vi "UHR-Fleezers Control (host) - 10.8.vi"() -> ()   [LabVIEW 2014] (continued)
    n2212 = Cluster To Array(cluster=w3125) -> (array=w3122:string[])
    n2213 = Bundle("APD 1", "APD 2") -> (w3310:cluster{string, string})  [unwired: 1 out]
    n2214 = Select(t=-1.0, s="Negate Y Axis", f=1.0) -> (s? t:f=w3066:dbl)
    n2215 = for "Trap Position" {
      tunnel: w3131 -> [w3506] mode=indexing
      tunnel: "Trap Pos. Disp. Downsample" -> [w3505]
      tunnel: w3047 -> [w3503]
      tunnel: w3127 -> [w3502]
      tunnel: w3126 -> [w3500]
      tunnel: w3122 -> [w3499] mode=indexing
      tunnel: [w3498] -> w3036 mode=indexing
      tunnel: w3081 -> [w3496] mode=indexing
      tunnel: w3080 -> [w3494]
      tunnel: w3066 -> [w3493]
      n2216 = call "downsample 1D array - double.vi"("Ave N"=w3505, "Array In"=w3506) -> ("Array Out"=w3504:dbl[])  [unwired: 1 out]
      n2217 = Subtract(x=w3504, y=w3496) -> (x-y=w3497:dbl[])
      n2218 = Multiply(x=w3494, y=w3497) -> (x*y=w3495:dbl[])
      n2219 = Multiply(x=w3493, y=w3495) -> (x*y=w3492:dbl[])
      n2220 = Bundle By Name("Y"=w3492, "dt"=w3503, "t0"=w3502) -> (w3501:waveform(dbl))  [unwired: 1 out]
      n2221 = Set Waveform Attribute(5:w3499, 6:w3500, 7:w3501) -> (3:w3498:waveform(dbl))  [unwired: 1 in, 2 out]
    }
    n2222 = Cluster To Array(cluster=w3310) -> (array=w3307:string[])
    n2223 = for "APD" {
      tunnel: w3278 -> [w3846] mode=indexing
      tunnel: w3156 -> [w3854]
      tunnel: [w3850] -> w3163 mode=indexing
      tunnel: "APD Disp. Scale" -> [w3851]
      tunnel: w3126 -> [w3849]
      tunnel: w3307 -> [w3848] mode=indexing
      tunnel: "APD Disp. Downsample" -> [w3844]
      tunnel: [w3847] -> w3306
      workers-P: _ -> [_]
      tunnel: w3127 -> [w3843]
      n2224 = call "integrate 1D array interval - double.vi"("Ave N"=w3844, "Array In"=w3846) -> ("Array Out"=w3845:dbl[])  [unwired: 1 out]
      n2225 = Multiply(x=w3854, y=w3844) -> (x*y=w3847:dbl)
      n2226 = Divide(x=w3845, y=w3851) -> (x/y=w3852:dbl[])
      n2227 = Bundle By Name("t0"=w3843, "Y"=w3852, "dt"=w3847) -> (w3853:waveform(dbl))  [unwired: 1 out]
      n2228 = Set Waveform Attribute(5:w3848, 6:w3849, 7:w3853) -> (3:w3850:waveform(dbl))  [unwired: 1 in, 2 out]
    }
    "APD Display Period (s)" <- w3306
    n2229 = Reciprocal(x=w3306) -> (1/x=→"APD Display Freq. (Hz)":dbl)
    n2230 = local read "Display Period (s)"() -> (w3187:dbl)
    n2231 = Increment(x=w3289) -> (x+1=w3290:dbl)
    n2232 = To Double Precision Float(number=w3199) -> (double precision float=w3198:dbl[])
    n2233 = Index Array(array=w3036, index=0) -> (element=w3040:waveform(dbl))
    n2234 = Index Array(array=w3036, index=1) -> (element=w3035:waveform(dbl))
    n2235 = feedback #7(w3290) -> (w3293:dbl)
    n2236 = Select(t=0, s=w3280, f=w3293) -> (s? t:f=w3286:dbl)
    n2237 = Array Size(array=w3198) -> (size(s)=w3292:i32)
    n2238 = Add(x=w3292, y=w3286) -> (x+y=w3287:dbl)
    n2239 = Unbundle By Name(w3040) -> ("Y"=w3041:dbl[])
    n2240 = feedback #8(w3199) -> (w3276:void[])
    n2241 = Build Array (concatenate)(w3276, w3199) -> (w3273:void[])
    n2242 = feedback #9(w3143) -> (w3162:void[])
    n2243 = Divide(x="Bead Sep. Int. Time (s)", y=w3187) -> (x/y=w3076:dbl)
    n2244 = Build Array (concatenate)(w3162, w3143) -> (w3161:void[])
    n2245 = Add(x=w3041, y="FB Trap Pos Offset") -> (x+y=w3039:dbl[])
    "T1 x pos data" <- w3039
    n2246 = Greater?(x=w3287, y=w3289) -> (0:w3288:bool)
    n2247 = feedback #10(w3039) -> (w3078:dbl[])
    n2248 = Build Array (concatenate)(w3039, w3078) -> (w3077:dbl[])
    n2249 = Bundle By Name(cluster=w3040, "Y"=w3039) -> (w3038:waveform(dbl))
    n2250 = Select(t=w3286, s=w3288, f=w3287) -> (s? t:f=w3285:dbl)
    n2251 = feedback-in #7(w3285) -> ()
    n2252 = Array Size(array=w3273) -> (size(s)=w3270:i32)
    n2253 = Array Size(array=w3199) -> (size(s)=w3272:i32)
    n2254 = local read "MCL Scanning"() -> (w3283:bool)
    n2255 = local read "APD Integration Time (s)"() -> (w3170:dbl)
    n2256 = Bundle(w3038, w3035) -> (w3034:cluster{waveform(dbl), waveform(dbl)})  [unwired: 1 out]
    n2257 = Build Array (concatenate)(w3163, w3311) -> (w3165:waveform(dbl)[])
    "All Signals" <- w3165
    n2258 = Split 1D Array(array=w3077, index=w3076) -> (first subarray=w3070:dbl[])  [unwired: 1 out]
    n2259 = feedback-in #10(w3070) -> ()
    n2260 = Multiply(x=w3272, y="APD Ave N") -> (x*y=w3271:dbl)
    n2261 = Greater?(x=w3270, y=w3271) -> (0:w3274:bool)
    n2262 = Not(x=w3288) -> (.not. x?=w3282:bool)
    n2263 = Cluster To Array(cluster=w3034) -> (array=→"Trap Positions":waveform(dbl)[])
    n2264 = To Double Precision Float(number=w3143) -> (double precision float=w3142:dbl[])
    n2265 = call-poly <vilib>:"Mean.vi"("X"=w3070) -> ("mean"=w3069:dbl)  [unwired: 1 out]
    "Mean T1 Position (nm)" <- w3069
    n2266 = Subtract(x=w3070, y=w3069) -> (x-y=w3075:dbl[])
    n2267 = Square(x=w3075) -> (x^2=w3074:dbl[])
    n2268 = And(x=w3282, y=w3283) -> (x .and. y?=w3284:bool)
    n2269 = call-poly <vilib>:"Mean.vi"("X"=w3074) -> ("mean"=w3073:dbl)  [unwired: 1 out]
    n2270 = case shown="True" w3274 {
      tunnel: w3273 -> [w3626 w3633]
      tunnel: [w3626 w3631] -> w3216
      tunnel: w3271 -> [_ w3628]
      tunnel: w3270 -> [_ w3632]
      tunnel: w3161 -> [w3625 w3630]
      tunnel: [w3625 w3627] -> w3158
      frame False {
      }
      frame True {
        n2271 = Subtract(x=w3632, y=w3628) -> (x-y=w3629:dbl)
        n2272 = Array Subset(array=w3633, index=w3629, length=w3628) -> (w3631:void[])
        n2273 = Array Subset(array=w3630, index=w3629, length=w3628) -> (w3627:void[])
      }
    }
    n2274 = feedback-in #8(w3216) -> ()
    n2275 = feedback-in #9(w3158) -> ()
    n2276 = Square Root(x=w3073) -> (sqrt(x)=w3072:dbl)
    n2277 = Or(x=w3284, y=w3280) -> (x .or. y?=w3281:bool)
    n2278 = Equal?(x="Tab Control 6", y=T34."High Res Display") -> (x = y?=w3205:bool)
    n2279 = Multiply(x="APD Disp. Scale", y=w3163) -> (x*y=w3172:waveform(dbl)[])
    n2280 = Multiply(x=10.0, y=w3072) -> (x*y=→"Trap 1 Position RMS (A)":dbl)
    n2281 = Multiply(x="APD Disp. Downsample", y=w3170) -> (x*y=w3168:dbl)
    n2282 = Divide(x=w3172, y=w3168) -> (x/y=w3140:waveform(dbl)[])
    n2283 = case "For displaying the high resolution display (no downsampling)" shown="True" w3205 {
      tunnel: w3167 -> [_ w3526]
      frame False {
      }
      frame True {
        n2284 = Index Array(array=w3526, index="High Res. Display") -> (element=w3527:waveform(dbl))
        n2285 = call <vilib>:"Std Deviation and Variance.vi"("X"=w3527) -> ("mean"=w3534:dbl, "standard deviation"=w3539:dbl)  [unwired: 1 in, 1 out]
        "Mean Intensity" <- w3534
        "Sigma" <- w3539
        n2286 = Subtract(x=w3527, y=w3534) -> (x-y=w3533:waveform(dbl))
        n2287 = Select(t=w3533, s="Subtract mean", f=w3527) -> (s? t:f=→"1 Channel":waveform(dbl))
        n2288 = Divide(x=w3539, y=w3534) -> (x/y=→"Sigma/Mean":dbl)
        n2289 = feedback #11(1) -> (w3528:i32)
        n2290 = Greater Or Equal?(x=w3528, y="Slow mean N ave.") -> (x >= y?=w3541:bool)
        n2291 = Increment(x=w3528) -> (x+1=w3543:i32)
        n2292 = Select(t=1, s=w3541, f=w3543) -> (s? t:f=w3530:i32)
        n2293 = feedback-in #11(w3530) -> ()
        n2294 = feedback #12() -> (w3531:waveform(dbl))  [unwired: 1 out]
        n2295 = case shown="Default" w3528 {
          tunnel: [w3546 w3549] -> w3532
          tunnel: w3531 -> [w3548 _]
          tunnel: w3527 -> [w3547 w3549]
          frame Default {
            n2296 = call-poly <vilib>:"Append Waveforms.vi"("waveform B"=w3547, "waveform A"=w3548) -> ("waveform out"=w3546:waveform(dbl))  [unwired: 1 in, 8 out]
          }
          frame 1 {
          }
        }
        n2297 = feedback-in #12(w3532) -> ()
        n2298 = case shown="True" w3541 {
          tunnel: w3532 -> [_ w3545]
          frame False {
          }
          frame True {
            n2299 = call-poly <vilib>:"Mean.vi"("X"=w3545) -> ("mean"=→"Slow mean":dbl)  [unwired: 1 out]
          }
        }
      }
    }
    n2300 = Index Array(array=w3140, index=0) -> (element=w3150:waveform(dbl))
    n2301 = Index Array(array=w3140, index=1) -> (element=w3148:waveform(dbl))
    n2302 = case "For computing FFTs for display" shown="True" "Compute FFT" {
      tunnel: w3167 -> [_ w4240]
      frame False {
      }
      frame True {
        n2303 = Build Array("FFT 1 Choice 1", "FFT 1 Choice 2", "FFT 2 Choice 1", "FFT 2 Choice 2") -> (w4233:u16[])
        n2304 = Array Size(array=w4240) -> (size(s)=w4239:i32)
        n2305 = feedback-in #13(w4233) -> ()
        n2306 = feedback #13(u16[] [100, 100, 100, 100]) -> (w4234:u16[])
        n2307 = feedback-in #14("# Spectra to Ave.") -> ()
        n2308 = feedback #14("# Spectra to Ave.") -> (w4231:dbl)
        n2309 = Not Equal?(x="# Spectra to Ave.", y=w4231) -> (x != y?=w4230:bool)
        n2310 = Not Equal?(x=w4233, y=w4234) -> (x != y?=w4232:bool)
        n2311 = feedback #15(1.0) -> (w4217:dbl)
        n2312 = Compound Arithmetic op=OR("Reset FFT", w4232, w4230) -> (w4215:bool)
        n2313 = Select(t=1.0, s=w4215, f=w4217) -> (s? t:f=w4219:dbl)
        n2314 = Greater?(x=w4219, y="# Spectra to Ave.") -> (0:w4238:bool)
        n2315 = Increment(x=w4219) -> (x+1=w4218:dbl)
        n2316 = feedback-in #15(w4218) -> ()
        n2317 = local read "DMA Update Period (s)"() -> (w4213:dbl)
        n2318 = Multiply(x="# Spectra to Ave.", y=w4213) -> (x*y=→"Ave. Time (s)":dbl)
        n2319 = Build Array(cluster{"f0":dbl, "df":dbl, "magnitude":dbl[]} {"f0"=0.0, "df"=0.0, "magnitude"=[]} ("PSD")) -> (w4222:cluster{"f0":dbl, "df":dbl, "magnitude":dbl[]}[])
        n2320 = Build Array(w4222, w4222, w4222, w4222) -> (w4224:T45)
        n2321 = feedback #16(w4224) -> (w4229:T45)
        n2322 = for {
          N: 4 -> [_]
          tunnel: w4233 -> [w4262] mode=indexing
          tunnel: w4240 -> [w4263]
          tunnel: w4239 -> [w4265]
          tunnel: w4215 -> [w4258]
          tunnel: w4238 -> [w4257]
          tunnel: "# Spectra to Ave." -> [w4256]
          tunnel: [w4255] -> w4228 mode=indexing
          tunnel: w4229 -> [w4260] mode=indexing
          tunnel: [w4259] -> w4216 mode=indexing
          tunnel: w4219 -> [w4254]
          n2323 = Less?(x=w4262, y=w4265) -> (x < y?=w4264:bool)
          n2324 = Index Array(array=w4263, index=w4262) -> (element=w4261:waveform(dbl))
          n2325 = case shown="True" w4264 {
            tunnel: w4261 -> [_ w4282]
            tunnel: w4260 -> [w4267 w4280]
            tunnel: [w4267 w4268] -> w4259
            tunnel: w4258 -> [_ w4279]
            tunnel: w4257 -> [_ w4272]
            tunnel: w4256 -> [_ w4271]
            tunnel: [cluster{"f0":dbl, "df":dbl, "magnitude":dbl[]} {"f0"=0.0, "df"=0.0, "magnitude"=[]} ("PSD") w4273] -> w4255
            tunnel: w4254 -> [_ w4270]
            frame False {
            }
            frame True {
              n2326 = call <vilib>:"Std Deviation and Variance.vi"("X"=w4282) -> ("mean"=w4283:dbl)  [unwired: 1 in, 2 out]
              n2327 = Subtract(x=w4282, y=w4283) -> (x-y=w4281:waveform(dbl))
              n2328 = xnode "Spectral Measurements"("Signals"=w4281) -> ("PSD"=w4275:cluster{"f0":dbl, "df":dbl, "magnitude":dbl[]})  [unwired: 1 in, 1 out]
              n2329 = case shown="False" w4279 {
                tunnel: w4280 -> [w4292 _]
                tunnel: [w4288 w4297] -> w4268
                tunnel: w4275 -> [w4291 w4298]
                tunnel: w4272 -> [w4290 _]
                frame False {
                  n2330 = Build Array (concatenate)(w4292, w4291) -> (w4289:cluster{"f0":dbl, "df":dbl, "magnitude":dbl[]}[])
                  n2331 = case shown="True" w4290 {
                    tunnel: w4289 -> [w4293 w4296]
                    tunnel: [w4293 w4294] -> w4288
                    frame False {
                    }
                    frame True {
                      n2332 = Delete From Array(array=w4296, index=0) -> (array with subset deleted=w4294:cluster{"f0":dbl, "df":dbl, "magnitude":dbl[]}[])  [unwired: 1 in, 1 out]
                    }
                  }
                }
                frame True {
                  n2333 = Build Array(w4298) -> (w4297:cluster{"f0":dbl, "df":dbl, "magnitude":dbl[]}[])
                }
              }
              n2334 = for {
                tunnel: w4268 -> [w4287] mode=indexing
                tunnel: [w4286] -> w4278 mode=indexing
                workers-P: _ -> [_]
                n2335 = Unbundle By Name(w4287) -> ("magnitude"=w4286:dbl[])
              }
              n2336 = Transpose 2D Array(2D array=w4278) -> (transposed array=w4277:dbl[][])
              n2337 = for {
                tunnel: w4277 -> [w4285] mode=indexing
                tunnel: [w4284] -> w4276 mode=indexing
                workers-P: _ -> [_]
                n2338 = Add Array Elements(numeric array=w4285) -> (sum=w4284:dbl)
              }
              n2339 = Select(t=w4271, s=w4272, f=w4270) -> (s? t:f=w4269:dbl)
              n2340 = Divide(x=w4276, y=w4269) -> (x/y=w4274:dbl[])
              n2341 = Bundle By Name(cluster=w4275, "magnitude"=w4274) -> (w4273:cluster{"f0":dbl, "df":dbl, "magnitude":dbl[]})
            }
          }
        }
        n2342 = case shown="True" w4215 {
          tunnel: w4216 -> [w4247 w4253]
          tunnel: [w4247 w4248] -> w4214
          frame False {
          }
          frame True {
            n2343 = Array Subset(array=w4253, index (row)=0 ("index"), length (row)=4 ("length"), index (col)=0 ("index"), length (col)=1 ("length")) -> (w4248:T45)
          }
        }
        n2344 = feedback-in #16(w4214) -> ()
        n2345 = Split 1D Array(array=w4228, index=2) -> (first subarray=→"FFT 1":cluster{"f0":dbl, "df":dbl, "magnitude":dbl[]}[], second subarray=→"FFT 2":cluster{"f0":dbl, "df":dbl, "magnitude":dbl[]}[])
      }
    }
    n2346 = case "For plotting results of scanning MCL" shown="True" w3281 {
      tunnel: w3280 -> [_ w3666]
      tunnel: w3198 -> [_ w3762]
      tunnel: w3289 -> [_ _]
      tunnel: w3167 -> [_ w3736]
      tunnel: w3142 -> [_ w3667]
      tunnel: w3141 -> [_ w3640]
      frame False {
      }
      frame True {
        w3647 = u32 0 items=["Horizontal", "Vertical", "Central", "1st Diagonal", "2nd Diagonal"] ("Type of Symmetry")
        w3675 = u32 0 items=["Horizontal", "Vertical", "Central", "1st Diagonal", "2nd Diagonal"] ("Type of Symmetry")
        w3678 = u32 0 items=["Horizontal", "Vertical", "Central", "1st Diagonal", "2nd Diagonal"] ("Type of Symmetry")
        w3707 = u32 0 items=["Horizontal", "Vertical", "Central", "1st Diagonal", "2nd Diagonal"] ("Type of Symmetry")
        n2347 = Index Array(array=w3736, index=10) -> (element=w3742:waveform(dbl))
        n2348 = Index Array(array=w3736, index=11) -> (element=w3739:waveform(dbl))
        n2349 = local read "Cycles/step (MCL)"() -> (w3692:u64)
        n2350 = Index Array(array=w3736, index="Channel") -> (element=w3738:waveform(dbl))
        n2351 = Unbundle(w3640) -> ("New Image"=w3639:T2, "New Image"=w3638:T2, "New Image"=w3637:T2, "New Image"=w3636:T2)
        n2352 = Unbundle By Name(w3742) -> ("Y"=w3694:dbl[])
        n2353 = Unbundle By Name(w3739) -> ("Y"=w3696:dbl[])
        n2354 = Unbundle By Name(w3738) -> ("Y"=w3701:dbl[])
        n2355 = call "downsample 1D array - double.vi"("Ave N"=w3692, "Array In"=w3694) -> ("Array Out"=w3693:dbl[])  [unwired: 1 out]
        n2356 = call "downsample 1D array - double.vi"("Ave N"=w3692, "Array In"=w3696) -> ("Array Out"=w3695:dbl[])  [unwired: 1 out]
        n2357 = call "downsample 1D array - double.vi"("Ave N"=w3692, "Array In"=w3701) -> ("Array Out"=w3700:dbl[])  [unwired: 1 out]
        n2358 = feedback #17(w3762) -> (w3763:dbl[])
        n2359 = Build Array (concatenate)(w3763, w3762) -> (w3744:dbl[])
        n2360 = feedback #18(w3667) -> (w3669:dbl[])
        n2361 = Build Array (concatenate)(w3669, w3667) -> (w3668:dbl[])
        n2362 = local read "Scan steps (MCL)"() -> (w3649:u64)
        n2363 = Select(t=w3762, s=w3666, f=w3744) -> (s? t:f=w3748:dbl[])
        n2364 = feedback-in #17(w3748) -> ()
        n2365 = Select(t=w3667, s=w3666, f=w3668) -> (s? t:f=w3650:dbl[])
        n2366 = feedback-in #18(w3650) -> ()
        n2367 = local read "Scan lines (y)"() -> (w3635:u64)
        n2368 = local read "N APD Samp/step"() -> (w3651:dbl)
        n2369 = feedback #19(w3693) -> (w3750:dbl[])
        n2370 = Build Array (concatenate)(w3750, w3693) -> (w3741:dbl[])
        n2371 = feedback #20(w3700) -> (w3760:dbl[])
        n2372 = Build Array (concatenate)(w3760, w3700) -> (w3759:dbl[])
        n2373 = feedback #21(w3695) -> (w3752:dbl[])
        n2374 = Build Array (concatenate)(w3752, w3695) -> (w3753:dbl[])
        n2375 = Select(t=w3693, s=w3666, f=w3741) -> (s? t:f=w3697:dbl[])
        n2376 = feedback-in #19(w3697) -> ()
        n2377 = Select(t=w3700, s=w3666, f=w3759) -> (s? t:f=w3699:dbl[])
        n2378 = feedback-in #20(w3699) -> ()
        n2379 = Select(t=w3695, s=w3666, f=w3753) -> (s? t:f=w3698:dbl[])
        n2380 = feedback-in #21(w3698) -> ()
        n2381 = Multiply(x=w3649, y=u64 2) -> (x*y=w3634:u64)
        n2382 = call "integrate 1D array interval - double.vi"("Ave N"=w3651, "Array In"=w3650) -> ("Array Out"=w3662:dbl[])  [unwired: 1 out]
        n2383 = call "integrate 1D array interval - double.vi"("Ave N"=w3651, "Array In"=w3748) -> ("Array Out"=w3747:dbl[])  [unwired: 1 out]
        n2384 = Array Size(array=w3662) -> (size(s)=w3663:i32)
        n2385 = Array Size(array=w3747) -> (size(s)=w3749:i32)
        n2386 = Multiply(x=w3635, y=w3634) -> (x*y=w3665:u64)
        n2387 = Multiply(x=w3635, y=w3634) -> (x*y=w3757:u64)
        n2388 = call-poly <vilib>:"Mean.vi"("X"=w3697) -> ("mean"=w3681:dbl)  [unwired: 1 out]
        n2389 = Subtract(x=w3665, y=w3663) -> (x-y=w3656:u64)
        n2390 = call-poly <vilib>:"Mean.vi"("X"=w3699) -> ("mean"=w3686:dbl)  [unwired: 1 out]
        n2391 = call-poly <vilib>:"Mean.vi"("X"=w3698) -> ("mean"=w3684:dbl)  [unwired: 1 out]
        n2392 = call-poly <vilib>:"Mean.vi"("X"=w3662) -> ("mean"=w3653:dbl)  [unwired: 1 out]
        n2393 = Subtract(x=w3757, y=w3749) -> (x-y=w3691:u64)
        n2394 = call-poly <vilib>:"Mean.vi"("X"=w3747) -> ("mean"=w3688:dbl)  [unwired: 1 out]
        n2395 = Initialize Array(1.0 ("element"), w3656) -> (w3652:dbl[])
        n2396 = Initialize Array(1.0 ("element"), w3691) -> (w3682:dbl[])
        n2397 = Multiply(x=w3652, y=w3653) -> (x*y=w3654:dbl[])
        n2398 = Multiply(x=w3682, y=w3684) -> (x*y=w3685:dbl[])
        n2399 = Multiply(x=w3682, y=w3686) -> (x*y=w3687:dbl[])
        n2400 = Multiply(x=w3682, y=w3681) -> (x*y=w3683:dbl[])
        n2401 = Multiply(x=w3682, y=w3688) -> (x*y=w3689:dbl[])
        n2402 = Build Array (concatenate)(w3697, w3683) -> (w3751:dbl[])
        n2403 = Build Array (concatenate)(w3699, w3687) -> (w3755:dbl[])
        n2404 = Build Array (concatenate)(w3698, w3685) -> (w3754:dbl[])
        n2405 = Build Array (concatenate)(w3662, w3654) -> (w3664:dbl[])
        n2406 = Build Array (concatenate)(w3747, w3689) -> (w3756:dbl[])
        n2407 = Reshape Array(w3751, w3635, w3634) -> (w3717:dbl[][])
        n2408 = Reshape Array(w3664, w3635, w3634) -> (w3660:dbl[][])
        n2409 = Reshape Array(w3755, w3635, w3634) -> (w3709:dbl[][])
        n2410 = Reshape Array(w3754, w3635, w3634) -> (w3724:dbl[][])
        n2411 = Reshape Array(w3756, w3635, w3634) -> (w3734:dbl[][])
        n2412 = Array Subset(array=w3724, index (col)=0 ("index"), length (col)=w3649) -> (w3729:dbl[][])  [unwired: 2 in]
        n2413 = Array Subset(array=w3724, index (col)=w3649) -> (w3727:dbl[][])  [unwired: 3 in]
        n2414 = Array Subset(array=w3709, index (col)=0 ("index"), length (col)=w3649) -> (w3715:dbl[][])  [unwired: 2 in]
        n2415 = Array Subset(array=w3709, index (col)=w3649) -> (w3713:dbl[][])  [unwired: 3 in]
        n2416 = Array Subset(array=w3660, index (col)=0 ("index"), length (col)=w3649) -> (w3659:dbl[][])  [unwired: 2 in]
        n2417 = Array Subset(array=w3660, index (col)=w3649) -> (w3657:dbl[][])  [unwired: 3 in]
        n2418 = Array Subset(array=w3734, index (col)=0 ("index"), length (col)=w3649) -> (w3733:dbl[][])  [unwired: 2 in]
        n2419 = Array Subset(array=w3734, index (col)=w3649) -> (w3731:dbl[][])  [unwired: 3 in]
        n2420 = Array Subset(array=w3717, index (col)=0 ("index"), length (col)=w3649) -> (w3722:dbl[][])  [unwired: 2 in]
        n2421 = Array Subset(array=w3717, index (col)=w3649) -> (w3720:dbl[][])  [unwired: 3 in]
        n2422 = for {
          tunnel: w3729 -> [w3771] mode=indexing
          tunnel: [w3770] -> w3728 mode=indexing
          workers-P: _ -> [_]
          n2423 = Reverse 1D Array(array=w3771) -> (reversed array=w3770:dbl[])
        }
        n2424 = for {
          tunnel: w3715 -> [w3767] mode=indexing
          tunnel: [w3766] -> w3714 mode=indexing
          workers-P: _ -> [_]
          n2425 = Reverse 1D Array(array=w3767) -> (reversed array=w3766:dbl[])
        }
        n2426 = for {
          tunnel: w3659 -> [w3765] mode=indexing
          tunnel: [w3764] -> w3658 mode=indexing
          workers-P: _ -> [_]
          n2427 = Reverse 1D Array(array=w3765) -> (reversed array=w3764:dbl[])
        }
        n2428 = for {
          tunnel: w3733 -> [w3773] mode=indexing
          tunnel: [w3772] -> w3732 mode=indexing
          workers-P: _ -> [_]
          n2429 = Reverse 1D Array(array=w3773) -> (reversed array=w3772:dbl[])
        }
        n2430 = for {
          tunnel: w3722 -> [w3769] mode=indexing
          tunnel: [w3768] -> w3721 mode=indexing
          workers-P: _ -> [_]
          n2431 = Reverse 1D Array(array=w3769) -> (reversed array=w3768:dbl[])
        }
        n2432 = Index Array(array=w3734, index (row)=0) -> (element=→"Waveform Graph":dbl[])  [unwired: 1 in]
        n2433 = Add(x=w3728, y=w3727) -> (x+y=w3726:dbl[][])
        n2434 = Add(x=w3714, y=w3713) -> (x+y=w3712:dbl[][])
        n2435 = Add(x=w3658, y=w3657) -> (x+y=w3642:dbl[][])
        n2436 = Add(x=w3732, y=w3731) -> (x+y=w3706:dbl[][])
        n2437 = Add(x=w3721, y=w3720) -> (x+y=w3719:dbl[][])
        n2438 = Divide(x=w3712, y=2) -> (x/y=w3710:dbl[][])
        n2439 = Divide(x=w3726, y=2) -> (x/y=w3671:dbl[][])
        n2440 = Divide(x=w3719, y=2) -> (x/y=w3673:dbl[][])
        n2441 = To Single Precision Float(number=w3706) -> (single precision float=w3705:sgl[][])
        n2442 = Transpose 2D Array(2D array=w3710) -> (transposed array=→"Data map":dbl[][])
        n2443 = To Single Precision Float(number=w3642) -> (single precision float=w3646:sgl[][])
        n2444 = To Single Precision Float(number=w3671) -> (single precision float=w3677:sgl[][])
        n2445 = To Single Precision Float(number=w3673) -> (single precision float=w3674:sgl[][])
        n2446 = call "IMAQ ArrayToImage"("Image Pixels (Float)"=w3705, "Image"=w3639) -> ("Image Out"=w3708:T2)  [unwired: 8 in, 1 out]
        n2447 = call "IMAQ ArrayToImage"("Image Pixels (Float)"=w3646, "Image"=w3638) -> ("Image Out"=w3648:T2)  [unwired: 8 in, 1 out]
        n2448 = call "IMAQ ArrayToImage"("Image Pixels (Float)"=w3677, "Image"=w3637) -> ("Image Out"=w3679:T2)  [unwired: 8 in, 1 out]
        n2449 = call "IMAQ ArrayToImage"("Image Pixels (Float)"=w3674, "Image"=w3636) -> ("Image Out"=w3676:T2)  [unwired: 8 in, 1 out]
        n2450 = call "IMAQ Symmetry"("Type of Symmetry"=w3707, "Image Src"=w3708) -> ("Image Dst Out"=w3703:T2)  [unwired: 3 in, 1 out]
        n2451 = call "IMAQ Symmetry"("Type of Symmetry"=w3647, "Image Src"=w3648) -> ("Image Dst Out"=w3644:T2)  [unwired: 3 in, 1 out]
        n2452 = call "IMAQ Symmetry"("Type of Symmetry"=w3678, "Image Src"=w3679) -> ("Image Dst Out"=→"Detection Laser X":T2)  [unwired: 3 in, 1 out]
        n2453 = call "IMAQ Symmetry"("Type of Symmetry"=w3675, "Image Src"=w3676) -> ("Image Dst Out"=→"Detection Laser Y":T2)  [unwired: 3 in, 1 out]
        n2454 = call "IMAQ Set Simple Calibration"("Calibration Axis Info"=T35 {"Origin Pixel"={"X"=0.0, "Y"=0.0}, "Angle Relative to Horizontal (deg)"=0.0, "Axis Reference"=0}, "Grid Descriptor"=T36 {"X Step"=0.3, "Y Step"=0.3, "Unit"=enum."Undefined"}, "Image"=w3703) -> ("Calibrated Image"=→"APD 1":T2)  [unwired: 7 in, 1 out]
        n2455 = call "IMAQ Set Simple Calibration"("Calibration Axis Info"=T35 {"Origin Pixel"={"X"=0.0, "Y"=0.0}, "Angle Relative to Horizontal (deg)"=0.0, "Axis Reference"=0}, "Grid Descriptor"=T36 {"X Step"=0.3, "Y Step"=0.3, "Unit"=enum."Undefined"}, "Image"=w3644) -> ("Calibrated Image"=→"APD 2":T2)  [unwired: 7 in, 1 out]
      }
    }
    n2456 = Subtract(x=w3148, y="APD 2 Offset") -> (x-y=w3145:waveform(dbl))
    n2457 = Subtract(x=w3150, y="APD 1 Offset") -> (x-y=w3146:waveform(dbl))
    n2458 = Index Array(array=w3165, index=3) -> (element=w3225:waveform(dbl))
    n2459 = Index Array(array=w3165, index=6) -> (element=w3222:waveform(dbl))
    n2460 = Build Array(w3146, w3145) -> (→"APD Chart":waveform(dbl)[])
    n2461 = Array Size(array=w3216) -> (size(s)=w3269:i32)
    n2462 = call <vilib>:"Std Deviation and Variance.vi"("X"=w3158) -> ("standard deviation"=w3157:dbl)  [unwired: 1 in, 2 out]
    n2463 = Add Array Elements(numeric array=w3158) -> (sum=w3160:dbl)
    n2464 = Add Array Elements(numeric array=w3216) -> (sum=w3279:dbl)
    n2465 = call <vilib>:"Std Deviation and Variance.vi"("X"=w3216) -> ("standard deviation"=w3215:dbl)  [unwired: 1 in, 2 out]
    n2466 = Divide(x="T1 offset_x (mV)", y=1000.0) -> (x/y=w3226:dbl)
    n2467 = Divide(x=w3157, y=w3156) -> (x/y=w3153:dbl)
    "Rate sigma (Hz) 2" <- w3153
    n2468 = Multiply(x=w3156, y=w3269) -> (x*y=w3159:dbl)
    "Int. Time (s)" <- w3159
    n2469 = Divide(x=w3160, y=w3159) -> (x/y=w3154:dbl)
    "APD 2 Rate (Hz)" <- w3154
    n2470 = Divide(x=w3279, y=w3159) -> (x/y=w3213:dbl)
    "APD 1 Rate (Hz)" <- w3213
    n2471 = Divide(x=w3215, y=w3156) -> (x/y=w3214:dbl)
    "Rate sigma (Hz)" <- w3214
    n2472 = Divide(x=w3153, y=w3154) -> (x/y=→"Sigma/Mean 2":dbl)
    n2473 = Divide(x=w3214, y=w3213) -> (x/y=→"Sigma/Mean":dbl)
    n2474 = feedback-in #22("Calibration") -> ()
    n2475 = feedback #22(u16 1 ("Calibration")) -> (w3246:u16)
    n2476 = Divide(x="T2 offset_x (mV)", y=1000.0) -> (x/y=w3224:dbl)
    n2477 = case shown="0, Default" "Calibration" {
      tunnel: "T1 alpha_x (nm/V)" -> [_ w3602 w3623]
      tunnel: "T1 kappa_x (pN/nm)" -> [_ _ w3613]
      tunnel: "T2 alpha_x (nm/V)" -> [_ w3601 w3621]
      tunnel: "T2 kappa_x (pN/nm)" -> [_ _ w3614]
      tunnel: w3225 -> [w3584 w3599 w3619]
      tunnel: w3222 -> [w3583 w3597 w3617]
      tunnel: [w3584 w3596 w3616] -> w3255
      tunnel: [w3583 w3595 w3615] -> w3254
      tunnel: ["T1 X (V)" ("Label.Text") "T1 X (nm)" ("Label.Text") "T1 X (pN)" ("Label.Text")] -> w3243
      tunnel: ["T2 X (V)" ("Label.Text") "T2 X (nm)" ("Label.Text") "T2 X (pN)" ("Label.Text")] -> w3242
      tunnel: ["Position (V)" ("Label.Text") "Position (nm)" ("Label.Text") "Force (pN)" ("Label.Text")] -> w3244
      tunnel: w3224 -> [_ w3587 w3606]
      tunnel: w3226 -> [_ w3590 w3608]
      tunnel: ["Mean (V)" ("Label.Text") "Mean (nm)" ("Label.Text") "Mean (pN)" ("Label.Text")] -> w3239
      tunnel: ["Difference (V)" ("Label.Text") "Difference (nm)" ("Label.Text") "Difference (pN)" ("Label.Text")] -> w3173
      frame 0, Default {
      }
      frame 1 {
        n2478 = Unbundle By Name(w3599) -> ("Y"=w3603:dbl[])
        n2479 = Unbundle By Name(w3597) -> ("Y"=w3588:dbl[])
        n2480 = Subtract(x=w3603, y=w3590) -> (x-y=w3591:dbl[])
        n2481 = Subtract(x=w3588, y=w3587) -> (x-y=w3589:dbl[])
        n2482 = Multiply(x=w3589, y=w3601) -> (x*y=w3598:dbl[])
        n2483 = Multiply(x=w3602, y=w3591) -> (x*y=w3600:dbl[])
        n2484 = Bundle By Name(cluster=w3597, "Y"=w3598) -> (w3595:waveform(dbl))
        n2485 = Bundle By Name(cluster=w3599, "Y"=w3600) -> (w3596:waveform(dbl))
      }
      frame 2 {
        n2486 = Unbundle By Name(w3619) -> ("Y"=w3624:dbl[])
        n2487 = Unbundle By Name(w3617) -> ("Y"=w3622:dbl[])
        n2488 = Subtract(x=w3622, y=w3606) -> (x-y=w3607:dbl[])
        n2489 = Subtract(x=w3624, y=w3608) -> (x-y=w3609:dbl[])
        n2490 = Compound Arithmetic op=MULTIPLY(w3607, w3621, w3614) -> (w3618:dbl[])
        n2491 = Compound Arithmetic op=MULTIPLY(w3613, w3623, w3609) -> (w3620:dbl[])
        n2492 = Bundle By Name(cluster=w3617, "Y"=w3618) -> (w3615:waveform(dbl))
        n2493 = Bundle By Name(cluster=w3619, "Y"=w3620) -> (w3616:waveform(dbl))
      }
    }
    n2494 = Not Equal?(x=w3246, y="Calibration") -> (x != y?=w3203:bool)
    n2495 = case shown="True" w3203 {
      tunnel: w3244 -> [_ w3577]
      tunnel: w3243 -> [_ w3576]
      tunnel: w3242 -> [_ w3575]
      tunnel: w3239 -> [_ w3574]
      tunnel: w3173 -> [_ w3573]
      frame False {
      }
      frame True {
        n2496 = property on="Force" class="WFChart (strict)"("YScale.NameLbl.Text"=w3577) -> ()  [unwired: 2 in, 2 out]
        n2497 = property on="T2 X" class="DigNum (strict)"("Caption.Text"=w3575) -> ()  [unwired: 2 in, 2 out]
        n2498 = property on="T1 X" class="DigNum (strict)"("Caption.Text"=w3576) -> ()  [unwired: 2 in, 2 out]
        n2499 = property on="Mean" class="DigNum (strict)"("Caption.Text"=w3574) -> ()  [unwired: 2 in, 2 out]
        n2500 = property on="Difference" class="DigNum (strict)"("Caption.Text"=w3573) -> ()  [unwired: 2 in, 2 out]
      }
    }
    n2501 = Unbundle By Name(w3225) -> ("Y"=w3228:dbl[])
    n2502 = Unbundle By Name(w3222) -> ("Y"=w3231:dbl[])
    n2503 = Subtract(x=w3228, y=w3226) -> (x-y=w3229:dbl[])
    n2504 = Subtract(x=w3231, y=w3224) -> (x-y=w3230:dbl[])
    n2505 = Multiply(x=w3230, y="T2 alpha_x (nm/V)") -> (x*y=w3014:dbl[])
    n2506 = Multiply(x="T1 alpha_x (nm/V)", y=w3229) -> (x*y=w3015:dbl[])
    n2507 = Not(x="Trap Trig. Fl.") -> (.not. x?=w3052:bool)
    n2508 = Multiply(x=w3254, y=-1.0) -> (x*y=w3233:waveform(dbl))
    n2509 = Subtract(x=w3015, y=w3014) -> (x-y=w3221:dbl[])
    n2510 = Unbundle By Name(w3254) -> ("Y"=w3192:dbl[])
    n2511 = Unbundle By Name(w3255) -> ("Y"=w3016:dbl[])
    n2512 = Negate(x=w3221) -> (-x=w3012:dbl[])
    n2513 = Build Array(w3255, w3233) -> (→"Force":waveform(dbl)[])
    n2514 = Subtract(x=w3012, y="Offset (nm)") -> (x-y=w3190:dbl[])
    n2515 = case shown="True" "Read Lateness and Rel Phase" {
      tunnel: w3032 -> [w3550 w3572]
      tunnel: w3031 -> [w3551 w3571]
      tunnel: [w3550 w3570] -> w3219
      tunnel: [w3551 w3569] -> w3218
      frame False {
      }
      frame True {
        n2516 = xnode "Read/Write Control"("FPGA VI Reference In"=w3572, "error in"=w3571) -> ("FPGA VI Reference Out"=w3570:T19, "error out"=w3569:errorcluster, "GI Relative phase"=→"GI relative phase", "Relative phase"=→"Relative phase (AI1)", "AI Late Counter"=→"Late Counter (AI1)", "GI Late Counter"=→"GI Late Counter", "MCL Late Counter"=→"MCL Late Counter", "MCL Relative Phase"=→"Relative Phase (MCL)", "APD Acq Relative Phase"=→"APD Acq Relative Phase", "APD 1 Gate Relative Phase"=→"APD 1 Gate Relative Phase", "APD 2 Gate Relative Phase"=→"APD 2 Gate Relative Phase", "APD Acq Late Counter"=→"APD Acq Late Counter", "APD 1 Gate Late Counter"=→"APD 1 Gate Late Counter", "APD 2 Gate Late Counter"=→"APD 2 Gate Late Counter", "Green FB Relative Phase"=→"Relative phase (Green FB)", "GI Relative phase 2"=→"GI relative phase 2", "GI Late Counter 2"=→"GI Late Counter 2", "Trap Pos FIFO Timeout"=→"Trap Pos FIFO Timeout", "Trap AI FIFO Timeout"=→"Trap AI FIFO Timeout")
      }
    }
    n2517 = call-poly <vilib>:"Mean.vi"("X"=w3192) -> ("mean"=w3018:dbl)  [unwired: 1 out]
    "T2 X" <- w3018
    n2518 = Negate(x=w3192) -> (-x=w3193:dbl[])
    n2519 = call-poly <vilib>:"Mean.vi"("X"=w3016) -> ("mean"=w3019:dbl)  [unwired: 1 out]
    "T1 X" <- w3019
    n2520 = Negate(x=w3018) -> (-x=w3017:dbl)
    n2521 = Bundle By Name(cluster=w3225, "Y"=w3190) -> (w3164:waveform(dbl))
    "Bead Separation" <- w3164
    n2522 = Add(x=w3016, y=w3193) -> (x+y=w3194:dbl[])
    n2523 = Add(x=w3019, y=w3017) -> (x+y=w3241:dbl)
    n2524 = Subtract(x=w3019, y=w3017) -> (x-y=→"Difference":dbl)
    n2525 = Divide(x=w3194, y=2.0) -> (x/y=→"Vec Mean of T1 T2":dbl[])
    n2526 = Divide(x=w3241, y=2.0) -> (x/y=w3196:dbl)
    "Mean" <- w3196
    n2527 = feedback-in #23("Trap Trig. Fl.") -> ()
    n2528 = feedback #23("Trap Trig. Fl.") -> (w3050:bool)
    n2529 = And(x=w3052, y=w3050) -> (x .and. y?=w3051:bool)
    n2530 = case "If have just turned off triggering" shown="True" w3051 {
      tunnel: w3032 -> [_ w3385]
      tunnel: w3031 -> [_ w3384]
      frame False {
      }
      frame True {
        w3383 = FALSE ("FPGA Trap Trig")
        n2531 = xnode "Read/Write Control"("FPGA VI Reference In"=w3385, "error in"=w3384, "FPGA Trap Trig"=w3383) -> ("FPGA VI Reference Out"=w3382:T19, "error out"=w3381:errorcluster)
        n2532 = xnode "Read/Write Control"("FPGA VI Reference In"=w3382, "error in"=w3381, "TTrig?"=w3383) -> ()  [unwired: 2 out]
        n2533 = local write "Initializing"(FALSE ("Initializing")) -> ()
        n2534 = local write "Triggered"(FALSE ("Triggered")) -> ()
        n2535 = local write "Waiting"(FALSE ("Waiting")) -> ()
      }
    }
    n2536 = Not(x=w3050) -> (.not. x?=w3063:bool)
    n2537 = And(x="Trap Trig. Fl.", y=w3063) -> (x .and. y?=w3060:bool)
    n2538 = local read "Tether"() -> (w3197:bool)
    n2539 = Or(x=w3060, y="Reinitialize") -> (x .or. y?=w3046:bool)
    n2540 = feedback #24(w3056) -> (w3061:string)
    n2541 = Select(t=w3056, s=w3060, f=w3061) -> (s? t:f=w3055:string)
    n2542 = Select(t=w3056, s="Reinitialize", f=w3055) -> (s? t:f=w3054:string)
    n2543 = feedback #25(0) -> (w3058:i32)
    n2544 = feedback #26(w3190) -> (w3189:dbl[])
    n2545 = Build Array (concatenate)(w3190, w3189) -> (w3013:dbl[])
    n2546 = case "For determining if there is a tether still" shown="True" w3197 {
      tunnel: w3196 -> [_ w3509]
      frame False {
      }
      frame True {
        n2547 = Greater?(x="Lost Tether Alarm Threshold (pN)", y=w3509) -> (0:w3507:bool)
        n2548 = case shown="True" w3507 {
          frame False {
          }
          frame True {
            w3510 = FALSE ("Value (Signaling)")
            n2549 = flat-sequence {
              frame #0 {
                # "stop only if saving"
                n2550 = local read "Saving..."() -> (w3522:bool)
                n2551 = And(x=w3522, y="TA Cancel Save?") -> (x .and. y?=w3521:bool)
                n2552 = local write "Stop Saving"(w3521) -> ()
              }
              frame #1 {
                n2553 = case shown="True" "TA Green Off?" {
                  frame False {
                  }
                  frame True {
                    w3525 = FALSE ("Fl. Triggered...")
                    n2554 = local write "Fl. Triggered..."(w3525) -> ()
                    n2555 = property on="Green Laser ON/Interlacing" class="Bool (strict)"("Val(Sgnl)"=w3525) -> ()  [unwired: 2 in, 2 out]
                  }
                }
              }
            }
            n2556 = local read "Time tether formed"() -> (w3516:timestamp)
            n2557 = Get Date/Time In Seconds() -> (seconds since 1Jan1904=w3517:timestamp)
            n2558 = Subtract(x=w3517, y=w3516) -> (x-y=w3515:dbl)
            n2559 = Number To Decimal String(number=w3515) -> (decimal integer string=w3512:string)  [unwired: 1 out]
            n2560 = local read "Messages"() -> (w3519:string)
            n2561 = call <vilib>:"Beep.vi"() -> ()  [unwired: 3 in, 9 out]
            n2562 = Concatenate Strings("Lost tether (" ("Message to add"), w3512, " s)." ("string")) -> (w3514:string)
            n2563 = local write "Tether"(FALSE ("Tether")) -> ()
            n2564 = call "Update messages.vi"("Message to add"=w3514, "Old message string"=w3519) -> ("New message string"=w3518:string)
            n2565 = local write "Messages"(w3518) -> ()
            n2566 = local write "Dip for Protein"(w3510) -> ()
            n2567 = property on="Trap Pos. FB ON" class="Bool (strict)"("Val(Sgnl)"=w3510) -> ()  [unwired: 2 in, 2 out]
            n2568 = property on="Trap Trig. Fl." class="Bool (strict)"("Val(Sgnl)"=w3510) -> ()  [unwired: 2 in, 2 out]
          }
        }
      }
    }
    n2569 = case "For triggering actions based on the trap position (e.g., turning the excitation laser on if trap under feedback moves so far)" shown="True" "Trap Trig. Fl." {
      tunnel: w3041 -> [_ w3398]
      tunnel: w3054 -> [_ w3397]
      tunnel: ["" ("t") w3396] -> w3062
      tunnel: w3046 -> [_ w3395]
      tunnel: [0 ("t") w3394] -> w3059
      tunnel: w3058 -> [_ w3393]
      tunnel: w3032 -> [_ w3392]
      tunnel: w3031 -> [_ w3391]
      frame False {
      }
      frame True {
        n2570 = case shown="\"Wait for trigger\"" w3397 {
          tunnel: w3398 -> [w3415 _ _ w3463]
          tunnel: [w3412 w3444 "" ("t") w3466] -> w3396
          tunnel: w3395 -> [_ _ _ w3454]
          tunnel: [w3411 w3441 0 ("t") w3455] -> w3394
          tunnel: w3393 -> [_ w3443 _ w3461]
          tunnel: w3392 -> [w3400 w3438 _ w3457]
          tunnel: w3391 -> [w3399 w3437 _ w3456]
          frame "Wait for trigger" {
            n2571 = local read "Trap Trig. (FPGA)"() -> (w3403:bool)
            n2572 = Subtract(x=w3415, y="Mean T1 Position\nto compare (nm)") -> (x-y=w3408:dbl[])
            n2573 = call <vilib>:"Std Deviation and Variance.vi"("X"=w3408) -> ("mean"=→"mean":dbl, "standard deviation"=→"standard\ndeviation":dbl)  [unwired: 1 in, 1 out]
            n2574 = Array Max & Min(array=w3408) -> (max value=→"max value":dbl, min value=→"min value":dbl)  [unwired: 2 out]
            n2575 = Greater?(x=w3408, y="Threshold (nm)") -> (0:w3418:bool[])
            n2576 = case shown="True" w3403 {
              tunnel: w3400 -> [_ w3424]
              tunnel: w3399 -> [_ w3423]
              tunnel: [FALSE ("TTrig?") w3422] -> w3406
              frame False {
              }
              frame True {
                n2577 = xnode "Read/Write Control"("FPGA VI Reference In"=w3424, "error in"=w3423) -> ("TTrig?"=w3422)  [unwired: 2 out]
              }
            }
            n2578 = Or Array Elements(Boolean array=w3418) -> (logical OR=w3405:bool)
            n2579 = Select(t=w3406, s=w3403, f=w3405) -> (s? t:f=w3404:bool)
            n2580 = Not(x=w3403) -> (.not. x?=w3402:bool)
            n2581 = And(x=w3404, y=w3402) -> (x .and. y?=w3401:bool)
            n2582 = Select(t="Triggered", s=w3404, f="Wait for trigger") -> (s? t:f=w3412:string)
            n2583 = case shown="True" w3404 {
              tunnel: [0 0] -> w3411
              tunnel: w3400 -> [_ w3429]
              tunnel: w3399 -> [_ w3428]
              frame False {
                "Waiting" <- TRUE ("Waiting")
              }
              frame True {
                n2584 = xnode "Read/Write Control"("FPGA VI Reference In"=w3429, "error in"=w3428, "TTrig?"=FALSE) -> ()  [unwired: 2 out]
                n2585 = local read "Messages"() -> (w3432:string)
                n2586 = call <vilib>:"Beep.vi"() -> ()  [unwired: 12 in]
                n2587 = call "Update messages.vi"("Message to add"="Unwinding trigger.", "Old message string"=w3432) -> ("New message string"=w3433:string)
                n2588 = local write "Messages"(w3433) -> ()
                n2589 = local write "Waiting"(FALSE ("Waiting")) -> ()
                "Triggered" <- TRUE ("Triggered")
              }
            }
            n2590 = case "Only need to turn on laser if host triggered" shown="True" w3401 {
              frame False {
              }
              frame True {
                n2591 = property on="Green Laser ON/Interlacing" class="Bool (strict)"("Val(Sgnl)"=TRUE ("Value (Signaling)")) -> ()  [unwired: 2 in, 2 out]
              }
            }
          }
          frame "Triggered" {
            n2592 = local read "Trap Trig. (FPGA)"() -> (w3440:bool)
            n2593 = Increment(x=w3443) -> (x+1=w3441:i32)
            n2594 = Greater Or Equal?(x=w3441, y="Fl. ON time (n)") -> (x >= y?=w3439:bool)
            n2595 = Select(t="Wait for trigger", s=w3439, f="Triggered" ("t")) -> (s? t:f=w3444:string)
            n2596 = And(x=w3439, y=w3440) -> (x .and. y?=w3436:bool)
            n2597 = case shown="True" w3436 {
              tunnel: w3438 -> [_ w3448]
              tunnel: w3437 -> [_ w3447]
              frame False {
              }
              frame True {
                n2598 = xnode "Read/Write Control"("FPGA VI Reference In"=w3448, "error in"=w3447, "FPGA Trap Trig"=TRUE) -> ()  [unwired: 2 out]
              }
            }
            n2599 = case shown="True" w3439 {
              frame False {
              }
              frame True {
                w3450 = FALSE ("Value (Signaling)")
                n2600 = local write "Triggered"(w3450) -> ()
                n2601 = local write "Waiting"(TRUE ("Waiting")) -> ()
                n2602 = property on="Green Laser ON/Interlacing" class="Bool (strict)"("Val(Sgnl)"=w3450) -> ()  [unwired: 2 in, 2 out]
              }
            }
          }
          frame "Do nothing" {
          }
          frame "Initialize", Default {
            n2603 = Increment(x=w3461) -> (x+1=w3465:i32)
            n2604 = Select(t=1, s=w3454, f=w3465) -> (s? t:f=w3455:i32)
            n2605 = feedback #27(w3463) -> (w3469:dbl[])
            n2606 = Build Array (concatenate)(w3463, w3469) -> (w3462:dbl[])
            n2607 = Greater Or Equal?(x=w3455, y="Wait to get offset (n)") -> (x >= y?=w3458:bool)
            n2608 = Select(t=w3463, s=w3454, f=w3462) -> (s? t:f=w3464:dbl[])
            n2609 = feedback-in #27(w3464) -> ()
            n2610 = call-poly <vilib>:"Mean.vi"("X"=w3464) -> ("mean"=w3459:dbl)  [unwired: 1 out]
            n2611 = local write "Mean T1 Position\nto compare (nm)"(w3459) -> ()
            n2612 = case shown="True" w3454 {
              tunnel: w3457 -> [_ w3475]
              tunnel: w3456 -> [_ w3474]
              frame False {
              }
              frame True {
                w3471 = FALSE ("FPGA Trap Trig")
                n2613 = xnode "Read/Write Control"("FPGA VI Reference In"=w3475, "error in"=w3474, "FPGA Trap Trig"=w3471) -> ("FPGA VI Reference Out"=w3473:T19, "error out"=w3472:errorcluster)
                n2614 = xnode "Read/Write Control"("FPGA VI Reference In"=w3473, "error in"=w3472, "TTrig?"=w3471) -> ()  [unwired: 2 out]
              }
            }
            n2615 = Select(t="Wait for trigger", s=w3458, f="Initialize") -> (s? t:f=w3466:string)
            n2616 = case shown="True" w3458 {
              tunnel: w3459 -> [_ w3478]
              tunnel: w3457 -> [_ w3487]
              tunnel: w3456 -> [_ w3486]
              frame False {
                n2617 = local write "Waiting"(FALSE ("Waiting")) -> ()
                "Initializing" <- TRUE ("Initializing")
              }
              frame True {
                n2618 = local read "Threshold (nm)"() -> (w3490:dbl)
                n2619 = local read "AOM X Cal (nm/MHz)"() -> (w3489:dbl)
                n2620 = Add(x=w3478, y=w3490) -> (x+y=w3491:dbl)
                n2621 = Divide(x=w3491, y=w3489) -> (x/y=w3488:dbl)
                n2622 = call "IR AOM freq to word.vi"("Frequency In (MHz)"=w3488) -> ("Frequency Word Out (double)"=w3485:dbl)
                n2623 = local write "Initializing"(FALSE ("Initializing")) -> ()
                n2624 = local write "Waiting"(TRUE ("Waiting")) -> ()
                n2625 = To Quad Integer(1:w3485) -> (0:w3484:i64)
                n2626 = xnode "Read/Write Control"("FPGA VI Reference In"=w3487, "error in"=w3486, "FPGA TTrig Thresh"=w3484) -> ("FPGA VI Reference Out"=w3481:T19, "error out"=w3480:errorcluster)
                n2627 = xnode "Read/Write Control"("FPGA VI Reference In"=w3481, "error in"=w3480, "FPGA Trap Trig"=TRUE) -> ()  [unwired: 2 out]
              }
            }
          }
        }
      }
    }
    n2628 = feedback-in #24(w3062) -> ()
    n2629 = feedback-in #25(w3059) -> ()
    n2630 = Split 1D Array(array=w3013, index=w3076) -> (first subarray=w3186:dbl[])  [unwired: 1 out]
    n2631 = feedback-in #26(w3186) -> ()
    n2632 = call-poly <vilib>:"Mean.vi"("X"=w3186) -> ("mean"=w3185:dbl)  [unwired: 1 out]
    "Bead Mean (nm)" <- w3185
    n2633 = Subtract(x=w3186, y=w3185) -> (x-y=w3184:dbl[])
    n2634 = Square(x=w3184) -> (x^2=w3183:dbl[])
    n2635 = call-poly <vilib>:"Mean.vi"("X"=w3183) -> ("mean"=w3182:dbl)  [unwired: 1 out]
    n2636 = Square Root(x=w3182) -> (sqrt(x)=w3181:dbl)
    n2637 = Multiply(x=10.0, y=w3181) -> (x*y=→"RMS (Ang)":dbl)
    n2638 = xnode "Read/Write Control"("FPGA VI Reference In"=w3219, "error in"=w3218) -> ("FPGA VI Reference Out"=w3044:T19, "error out"=w3043:errorcluster, "AI2 Y Sum Set 1"=w3325, "AI2 Y Sum Set 2"=w3324, "AI1 X Set 1"=w3108, "AI1 X Set 2"=w3107, "Trap Pos FB Int Signal"=→"Trap Pos FB Int Signal", "Trap Pos FB Int-Norm Signal"=→"Trap Pos FB Int-Norm Signal", "Trap Pos FB Action"=w3101, "Scanning"=→"AOD Scanning", "Scan I"=→"AOD Scan I", "Scanning MCL"=w3327, "Scan I (MCL)"=→"MCL Scan I", "Green FB Signals"=w3264, "TTrig Sig"=w3030, "TTrig Fin Thresh"=w3026)
    "MCL Scanning" <- w3327
    "Trap Pos FB Action" <- w3101
    n2639 = local read "FB Trig Integrate"() -> (w3024:u32)
    n2640 = Divide(x=w3030, y=w3024) -> (x/y=w3023:dbl)
    "TTrig Sig (Int)" <- w3023
    n2641 = Divide(x=w3026, y=w3024) -> (x/y=w3021:dbl)
    "TTrig Fin Thresh (Int)" <- w3021
    n2642 = local read "AOM X Cal (nm/MHz)"() -> (w3029:dbl)
    n2643 = local read "AI2 (V)"() -> (w3326:cluster{"Set 1":dbl, "Set 2":dbl})
    n2644 = Bundle By Name(cluster=w3326, "Set 1"=w3325, "Set 2"=w3324) -> (w3322:cluster{"Set 1":dbl, "Set 2":dbl})
    n2645 = Divide(x=w3101, y=327.67) -> (x/y=→"Action (%)":dbl)
    n2646 = local read "Trap X (AI1)"() -> (w3121:T10)
    n2647 = call "IR AOM word double to freq.vi"("Frequency Word In (double)"=w3021) -> ("Frequency Out (MHz)"=w3020:dbl)
    n2648 = call "IR AOM word double to freq.vi"("Frequency Word In (double)"=w3023) -> ("Frequency Out (MHz)"=w3022:dbl)
    n2649 = Divide(x=w3322, y=3276.7) -> (x/y=w3321:cluster{"Set 1":dbl, "Set 2":dbl})
    n2650 = Multiply(x=w3022, y=w3029) -> (x*y=w3028:dbl)
    "TTrig Sig (nm)" <- w3028
    n2651 = Multiply(x=w3020, y=w3029) -> (x*y=w3027:dbl)
    "TTrig Fin Thresh (nm)" <- w3027
    n2652 = local write "AI2 (V)"(w3321) -> ()
    n2653 = Bundle(cluster=w3121, "Trap 1"=w3108, "Trap 2"=w3107) -> (→"Trap X (AI1)":T10)
    n2654 = Bundle(w3028, w3027) -> (→"TTrig":cluster{dbl, dbl})  [unwired: 1 in]
    n2655 = Divide(x=w3264, y=3276.7) -> (x/y=w3260:dbl)
    n2656 = Unbundle By Name(w3260) -> ("Green FB Ch 0"=w3263, "Green FB Ch 1"=w3262, "Green FB Ch 2"=w3261)
    n2657 = Divide(x=w3263, y=w3261) -> (x/y=w3259:dbl)
    n2658 = Divide(x=w3262, y=w3261) -> (x/y=w3258:dbl)
    n2659 = flat-sequence "To save data" {
      tunnel: [w4346] -> w3345
      tunnel: [w4347] -> w3344
      tunnel: w3295 -> [w4340]
      tunnel: w3049 -> [w4344]
      tunnel: ["Save Calibration"] -> w3318
      tunnel: w3315 -> [w4343]
      tunnel: [w4336] -> w3314
      tunnel: [w4333] -> w3313
      tunnel: [w4330] -> w3312
      tunnel: w3294 -> [w4332]
      tunnel: w3201 -> [w4326]
      tunnel: [w4326] -> w3200
      tunnel: ["Start Saving"] -> w3166
      tunnel: [w4320] -> w3089
      tunnel: [w4319] -> w3088
      tunnel: w3345 -> [w4581]
      tunnel: w3344 -> [w4580]
      tunnel: w3090 -> [w4579]
      tunnel: w3318 -> [w4578]
      tunnel: w3314 -> [w4576]
      tunnel: w3313 -> [w4575]
      tunnel: w3312 -> [w4574]
      tunnel: w3175 -> [w4573]
      tunnel: w3211 -> [w4572]
      tunnel: w3200 -> [w4571]
      tunnel: w3166 -> [w4570]
      tunnel: w3164 -> [w4569]
      tunnel: w3140 -> [w4568]
      tunnel: w3089 -> [w4567]
      tunnel: w3088 -> [w4566]
      tunnel: w3087 -> [w4565]
      frame #0 {
        n2660 = Or(x="Save N Sets", y="Start Saving") -> (x .or. y?=w4327:bool)
        n2661 = To Double Precision Float(number=w4343) -> (double precision float=w4337:dbl)
        n2662 = Build Array(w4327, "Save Calibration", w4340, w4332) -> (w4342:bool[])
        n2663 = Compound Arithmetic op=OR("Save Calibration", w4340, w4327, w4332) -> (w4345:bool)
        n2664 = Boolean Array To Number(Boolean array=w4342) -> (number=w4339:u32)
        n2665 = feedback #28(FALSE ("Save APD Data\nwith Trap Data")) -> (w4321:bool)
        n2666 = feedback #29(refnum<k0> refnum) -> (w4348:refnum<file>)
        n2667 = feedback #30(refnum<k0> refnum) -> (w4323:refnum<file>)
        n2668 = feedback #31(FALSE ("Save APD Data\nwith Trap Data")) -> (w4331:bool)
        n2669 = feedback #32(refnum<k0> refnum) -> (w4334:refnum<file>)
        n2670 = feedback #33(0) -> (w4350:i32)
        n2671 = feedback #34() -> (w4338:u32)  [unwired: 1 out]
        n2672 = case shown="True" w4345 {
          tunnel: [w4357 1] -> w4346
          tunnel: w4350 -> [w4359 _]
          tunnel: [w4358 w4377] -> w4347
          tunnel: w4348 -> [w4358 _]
          tunnel: w4344 -> [_ w4397]
          tunnel: w4337 -> [_ w4395]
          tunnel: w4339 -> [_ w4398]
          tunnel: [w4356 w4376] -> w4336
          tunnel: w4338 -> [w4356 _]
          tunnel: [w4355 w4374] -> w4333
          tunnel: w4334 -> [w4355 _]
          tunnel: [w4354 w4373] -> w4330
          tunnel: w4331 -> [w4354 _]
          tunnel: "Start Saving" -> [_ w4371]
          tunnel: w4326 -> [_ w4370]
          tunnel: [w4353 w4361] -> w4319
          tunnel: w4323 -> [w4353 _]
          tunnel: [w4352 w4360] -> w4320
          tunnel: w4321 -> [w4352 _]
          frame False {
            n2673 = Increment(x=w4359) -> (x+1=w4357:i32)
          }
          frame True {
            w4367 = FALSE ("Start Saving")
            w4372 = 9.0  # File Version
            w4380 = FALSE ("prepend array or string size? (T)")
            w4378 = T24."big-endian, network order" ("byte order (0:big-endian, network order)")
            n2674 = local read "BD 1 Frequency 1 (MHz)"() -> (w4394:dbl)
            n2675 = local read "BD 2 Frequency 1 (MHz)"() -> (w4393:dbl)
            n2676 = local read "BD 1 Frequency 2 (MHz)"() -> (w4392:dbl)
            n2677 = local read "BD 2 Frequency 2 (MHz)"() -> (w4391:dbl)
            n2678 = local read "BD 1 Frequency 3 (MHz)"() -> (w4390:dbl)
            n2679 = local read "BD 2 Frequency 3 (MHz)"() -> (w4389:dbl)
            n2680 = Array Size(array=w4370) -> (size(s)=w4369:i32)
            n2681 = To Double Precision Float(number=w4369) -> (double precision float=w4368:dbl)
            n2682 = local write "Save Calibration"(w4367) -> ()
            n2683 = local write "Start Saving"(w4367) -> ()
            n2684 = Build Array("Save APD Data\nwith Trap Data", "Save Trap Pos. Data") -> (w4364:bool[])
            n2685 = Boolean Array To Number(Boolean array=w4364) -> (number=w4363:u32)
            n2686 = Build Array(w4394, w4393, w4392, w4391, w4390, w4389) -> (w4388:dbl[])
            n2687 = case shown="1, Default" w4398 {
              tunnel: w4397 -> [w4469 w4489 w4505 w4543]
              tunnel: w4368 -> [w4474 w4496 w4525 w4562]
              tunnel: w4395 -> [w4473 w4495 w4524 w4561]
              tunnel: [w4470 w4491 w4516 w4553] -> w4386
              tunnel: [w4461 "Cal sets to save" w4506 w4544] -> w4376
              tunnel: w4388 -> [w4471 w4492 w4518 w4555]
              tunnel: "Save APD Data\nwith Trap Data" -> [w4468 _ w4502 w4541]
              tunnel: [w4468 w4483 w4502 w4541] -> w4373
              tunnel: w4372 -> [w4464 w4484 w4500 w4539]
              tunnel: w4371 -> [w4463 _ _ _]
              tunnel: [w4454 w4483 w4499 w4529] -> w4360
              tunnel: "Save Trap Pos. Data" -> [w4454 _ w4499 w4529]
              tunnel: w4363 -> [w4453 _ w4498 w4528]
              frame 1, Default {
                # "timeseries"
                n2688 = case shown="True" "Profile" {
                  tunnel: [w4477 w4481] -> w4458
                  tunnel: [w4477 w4480] -> w4457
                  tunnel: [w4477 w4479] -> w4456
                  tunnel: [w4477 w4478] -> w4455
                  frame False {
                    w4477 = 0.0 ("f")
                  }
                  frame True {
                    n2689 = local read "Current Position"() -> (w4482:cluster{dbl, dbl, dbl})
                    n2690 = local read "Y change (mm)"() -> (w4478:dbl)
                    n2691 = Unbundle(w4482) -> (w4481:dbl, w4480:dbl, w4479:dbl)
                  }
                }
                n2692 = local read "Save ave N"() -> (w4476:dbl)
                n2693 = Multiply(x=w4476, y=w4469) -> (x*y=w4475:dbl)
                n2694 = To Double Precision Float(number=w4453) -> (double precision float=w4467:dbl)
                n2695 = Build Array(w4464, w4469, w4475, w4474, w4473, 0.0 ("f")) -> (w4472:dbl[])
                n2696 = Build Array(w4467, w4458, w4457, w4456, w4455) -> (w4465:dbl[])
                n2697 = Select(t=u32 4000000000, s=w4463, f="N sets to save") -> (s? t:f=w4461:u32)
                n2698 = Build Array (concatenate)(w4472, w4471, w4465) -> (w4470:dbl[])
              }
              frame 2 {
                w4486 = 0.0 ("f")
                w4483 = FALSE ("Save APD Data\nwith Trap Data")
                # "calibration"
                n2699 = Boolean To (0,1)(Boolean=w4483) -> (0, 1=w4488:i16)
                n2700 = To Double Precision Float(number=w4488) -> (double precision float=w4487:dbl)
                n2701 = Build Array(w4487, w4486, w4486, w4486, w4486) -> (w4485:dbl[])
                n2702 = Build Array(w4484, w4489, w4489, w4496, w4495, 1.0 ("t")) -> (w4493:dbl[])
                n2703 = Build Array (concatenate)(w4493, w4492, w4485) -> (w4491:dbl[])
                "Calibrating Trap..." <- TRUE ("Calibrating...")
              }
              frame 4 {
                w4503 = 0.0 ("f")
                # "scan dir (x/y = 0/1)"
                # "cycles/step"
                # "n scans (f/b)"
                # "steps"
                # "freq. range"
                # "AOD raster scan"
                n2704 = local read "Number of F/B Scans (AOD)"() -> (w4510:u16)
                n2705 = local read "Cycles/step (AOD)"() -> (w4512:u64)
                n2706 = local read "Scan Range (MHz)"() -> (w4515:dbl)
                n2707 = local read "Scan steps (AOD)"() -> (w4514:u64)
                n2708 = local read "Scan BD"() -> (w4522:bool)
                n2709 = local read "Save ave N"() -> (w4527:dbl)
                n2710 = Boolean To (0,1)(Boolean=w4522) -> (0, 1=w4521:i16)
                n2711 = To Double Precision Float(number=w4510) -> (double precision float=w4509:dbl)
                n2712 = To Double Precision Float(number=w4514) -> (double precision float=w4513:dbl)
                n2713 = To Double Precision Float(number=w4512) -> (double precision float=w4511:dbl)
                n2714 = To Double Precision Float(number=w4521) -> (double precision float=w4520:dbl)
                n2715 = Multiply(x=w4527, y=w4505) -> (x*y=w4526:dbl)
                n2716 = To Double Precision Float(number=w4498) -> (double precision float=w4504:dbl)
                n2717 = Build Array(w4504, w4503, w4503, w4503, w4503) -> (w4501:dbl[])
                n2718 = local read "N sets should be saved"() -> (w4507:dbl)
                n2719 = Build Array(w4520, w4515, w4513, w4511, w4509) -> (w4517:dbl[])
                n2720 = Build Array(w4500, w4505, w4526, w4525, w4524, 2.0 ("t")) -> (w4519:dbl[])
                n2721 = Round Toward +Infinity(x=w4507) -> (ceil(x): smallest int >= x=w4508:dbl)
                n2722 = Build Array (concatenate)(w4519, w4518, w4501, w4517) -> (w4516:dbl[])
                n2723 = To Unsigned Long Integer(number=w4508) -> (unsigned 32bit integer=w4506:u32)
              }
              frame 8 {
                w4536 = 0.0 ("f")
                # "MCL raster scan"
                n2724 = local read "Number of scans (MCL)"() -> (w4531:u64)
                n2725 = local read "Scan lines (y)"() -> (w4530:u64)
                n2726 = local read "2D or 1D Scan"() -> (w4533:bool)
                n2727 = local read "Scan Range (V)\n(of steps)"() -> (w4552:dbl)
                n2728 = local read "Fast Scan Dir"() -> (w4559:bool)
                n2729 = local read "Cycles/step (MCL)"() -> (w4549:u64)
                n2730 = local read "Scan steps (MCL)"() -> (w4551:u64)
                n2731 = Select(t=w4530, s=w4533, f=w4531) -> (s? t:f=w4532:u64)
                n2732 = Boolean To (0,1)(Boolean=w4533) -> (0, 1=w4535:i16)
                n2733 = local read "Save ave N"() -> (w4564:dbl)
                n2734 = local read "Initial X"() -> (w4538:dbl)
                n2735 = local read "Initial Y"() -> (w4537:dbl)
                n2736 = To Double Precision Float(number=w4535) -> (double precision float=w4534:dbl)
                n2737 = Boolean To (0,1)(Boolean=w4559) -> (0, 1=w4558:i16)
                n2738 = To Double Precision Float(number=w4532) -> (double precision float=w4547:dbl)
                n2739 = To Double Precision Float(number=w4551) -> (double precision float=w4550:dbl)
                n2740 = To Double Precision Float(number=w4549) -> (double precision float=w4548:dbl)
                n2741 = To Double Precision Float(number=w4558) -> (double precision float=w4557:dbl)
                n2742 = Multiply(x=w4564, y=w4543) -> (x*y=w4563:dbl)
                n2743 = To Double Precision Float(number=w4528) -> (double precision float=w4542:dbl)
                n2744 = local read "N sets should be saved (MCL)"() -> (w4545:dbl)
                n2745 = Build Array(w4542, w4534, w4536, w4536, w4536) -> (w4540:dbl[])
                n2746 = Build Array(w4557, w4552, w4550, w4548, w4547, w4538, w4537) -> (w4554:dbl[])
                n2747 = Build Array(w4539, w4543, w4563, w4562, w4561, 3.0 ("t")) -> (w4556:dbl[])
                n2748 = Round Toward +Infinity(x=w4545) -> (ceil(x): smallest int >= x=w4546:dbl)
                n2749 = Build Array (concatenate)(w4556, w4555, w4540, w4554) -> (w4553:dbl[])
                n2750 = To Unsigned Long Integer(number=w4546) -> (unsigned 32bit integer=w4544:u32)
              }
            }
            n2751 = local read "Index"() -> (w4403:dbl)
            n2752 = call "Create new save file.vi"("Insert"="", "Ext"=".dat", "Index In"=w4403) -> ("Path Out"=w4362:path, "Index Out"=w4375:dbl)
            n2753 = local write "Save file name"(w4362) -> ()
            n2754 = local write "Index"(w4375) -> ()
            n2755 = local write "Save index"(w4375) -> ()
            n2756 = Array Size(array=w4386) -> (size(s)=w4387:i32)
